vi "Calc_angles_and_ratios.v1.vi"(7 "COS ratio (TO/FROM) - internal":dbl=0.99999, 11 "Angle FROM deg (ext)":dbl=7.5) -> (0 "V at angle TO":dbl=209.7885634804175, 1 "V at angle FROM":dbl=209.7885634804175, 2 "Cos  FROM  (internal)":dbl=0.9993007047883986, 3 "Angle TO  deg (ext)":dbl=6.959125577482326)   [LabVIEW 2010]
panel:
  out "CosTO (internal)":dbl=0.9993007047883986
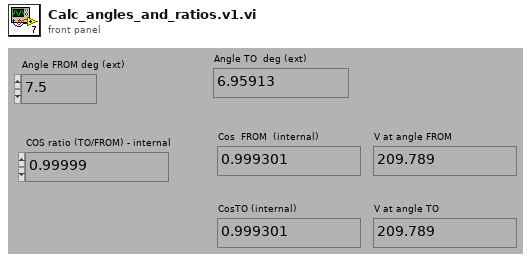
[diagram p1: front panel]
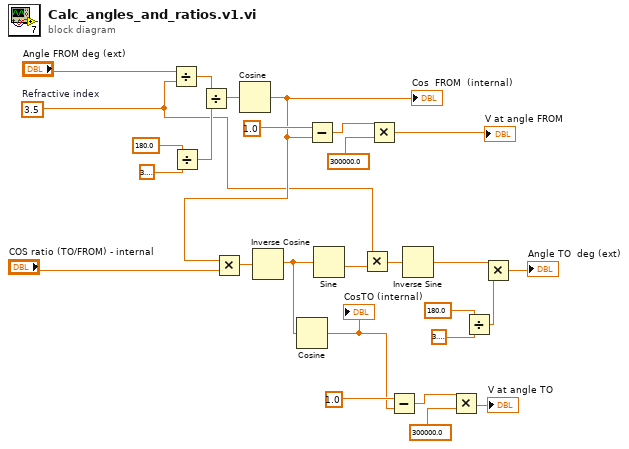
[diagram p0: block diagram]
diagram:
  w16 = sgl 3.5  # Refractive index
  n1 = Divide(x="Angle FROM deg (ext)", y=w16) -> (x/y=w19:dbl)
  n2 = Divide(x=sgl 180.0, y=3.141592653589793) -> (x/y=w25:dbl)
  n3 = Divide(x=w19, y=w25) -> (x/y=w24:dbl)
  n4 = Cosine(x=w24) -> (cos(x)=w18:dbl)
  "Cos  FROM  (internal)" <- w18
  n5 = Multiply(x=w18, y="COS ratio (TO/FROM) - internal") -> (x*y=w4:dbl)
  n6 = Inverse Cosine(1:w4) -> (0:w2:dbl)
  n7 = Cosine(x=w2) -> (cos(x)=w1:dbl)
  "CosTO (internal)" <- w1
  n8 = Subtract(x=sgl 1.0, y=w18) -> (x-y=w21:dbl)
  n9 = Sine(x=w2) -> (sin(x)=w17:dbl)
  n10 = Multiply(x=w16, y=w17) -> (x*y=w15:dbl)
  n11 = Multiply(x=w21, y=sgl 300000.0) -> (x*y=→"V at angle FROM":dbl)
  n12 = Subtract(x=sgl 1.0, y=w1) -> (x-y=w8:dbl)
  n13 = Inverse Sine(1:w15) -> (0:w12:dbl)
  n14 = Multiply(x=w8, y=sgl 300000.0) -> (x*y=→"V at angle TO":dbl)
  n15 = Divide(x=sgl 180.0, y=3.141592653589793) -> (x/y=w11:dbl)
  n16 = Multiply(x=w12, y=w11) -> (x*y=→"Angle TO  deg (ext)":dbl)
